vi "Main.vi"(11 "Module Admin":refnum<class "Delacor_lib_QMH_Module Admin.lvclass">) -> ()   [LabVIEW 2021, in "Caption Property Panel.lvlib"]
doc: "This template is based off of the Queued Message Handler design pattern and the Queued Message Handler project template that ships with LabVIEW.\n\nThe main difference is that the queue is private to this module and communication between modules is performed via Broadcast and Request events.\n\nRequest events are wrapped in public API methods and are handled in the Event Handling Loop (EHL) of this VI. Any module can register for Broadcast events sent by this module. The EHL generates messages based on user interface actions.\n\nThe Message Handling Loop (MHL) processes messages generated by the EHL, or by other messages. The messages are string values, so new messages can be added easily to the Message Cases case structure in the MHL. Each message cluster can also provide an optional value for Message Data, which is a variant that can be converted to whatever message-specific data is required.\n_____\nBased on DQMH Project Template 6.0.0.91."
uses:
  Caption Property Panel.lvlib
  <vilib>/Delacor/Delacor QMH/Libraries/Module Admin_class/Delacor_lib_QMH_Module Admin.lvclass
  Module Data--cluster.ctl
  <vilib>/Delacor/Delacor QMH/Libraries/Message Queue_class/Delacor_lib_QMH_Message Queue.lvclass/Delacor_lib_QMH_Message Queue.ctl
  Stop Argument--cluster.ctl
  <vilib>/Delacor/Delacor QMH/Libraries/Module Admin_class/Delacor_lib_QMH_Module Admin.lvclass/Delacor_lib_QMH_Module Admin.ctl
  Initialize Property Value Argument--cluster.ctl
  Load Panel Argument--cluster.ctl
  <vilib>/Utility/miscctls.llb/LVPointTypeDef.ctl
  <vilib>/Delacor/Delacor QMH/Libraries/Message Queue_class/Delacor_lib_QMH_Enqueue Message (Single).vi
  <vilib>/Delacor/Delacor QMH/Libraries/Module Admin_class/Delacor_lib_QMH_Get External Launch.vi
  <vilib>/Utility/error.llb/Error Cluster From Error Code.vi
  <vilib>/ErrorRing/Error Ring.xnode
  <vilib>/Delacor/Delacor QMH/Libraries/Message Queue_class/Delacor_lib_QMH_Message Queue.lvclass
panel:
  in  "Caption":string
  out "error out":errorcluster
  out "Status":string
  in  "Simulate MHL Error":bool
  in  "Simulate EHL Error":bool
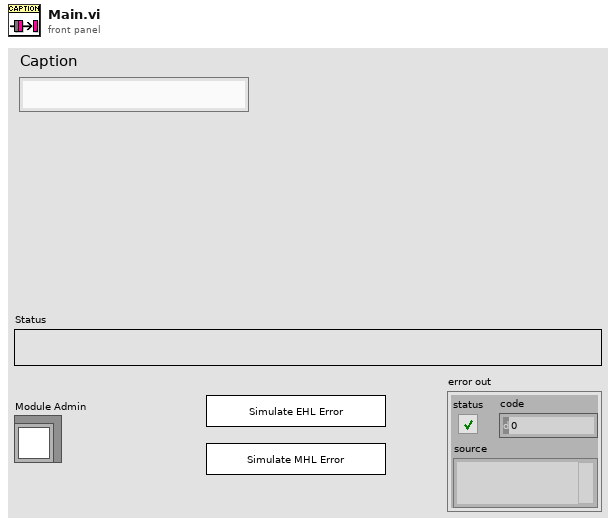
[diagram p1: front panel]
types:
  T1 = typedef "Caption Property Panel.lvlib/Request Events--cluster.ctl" = cluster{"Stop Module":refnum<user-event>, "Show Panel":refnum<user-event>, "Hide Panel":refnum<user-event>, "Get Module Execution Status":refnum<user-event>, "Show Diagram":refnum<user-event>, "Initialize Property Value":refnum<user-event>, "Load Panel":refnum<user-event>}
  T2 = typedef "Caption Property Panel.lvlib/Module Data--cluster.ctl" = cluster{"Status":string}
  T3 = enum32{"invalid lock state", "Not Locked", "Locked (No Password)", "Password-protected"}
  T4 = typedef "Caption Property Panel.lvlib/Stop Argument--cluster.ctl" = cluster{"Origin":string, "Exit via Stop Module Req?":bool, "Wait for Module to stop?":bool}
  T5 = typedef "Caption Property Panel.lvlib/Initialize Property Value Argument--cluster.ctl" = cluster{"Property values":variant[]}
  T6 = typedef "Caption Property Panel.lvlib/Load Panel Argument--cluster.ctl" = cluster{"SubPnl Refnum":refnum<vi>}
  T7 = typedef "LVPointTypeDef.ctl" = cluster{"Horizontal":i16, "Vertical":i16}
  T8 = enum32{"Invalid", "Standard", "Closed", "Hidden", "Minimized", "Maximized"}
  T9 = cluster{"Property value":string, "Variant data":variant}
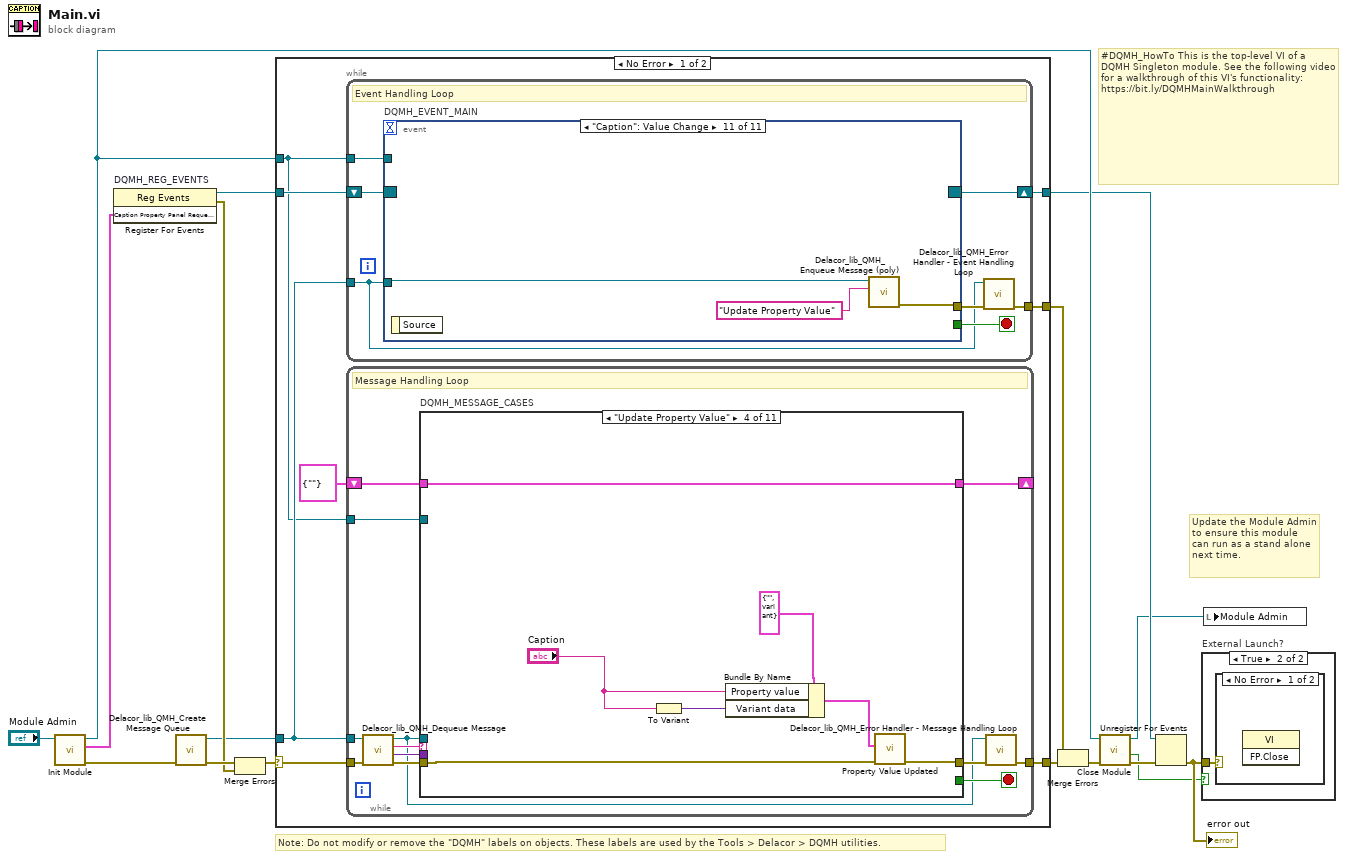
[diagram p0: block diagram]
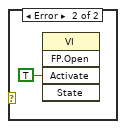
[diagram p3: hidden frame]
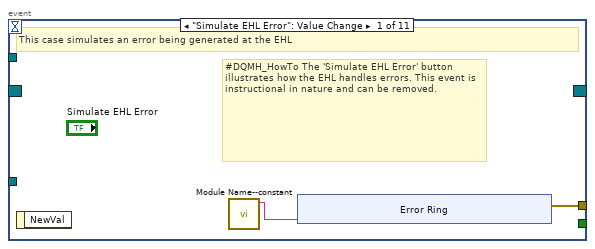
[diagram p4: hidden frame]
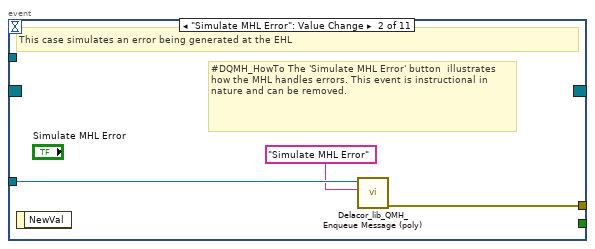
[diagram p5: hidden frame]
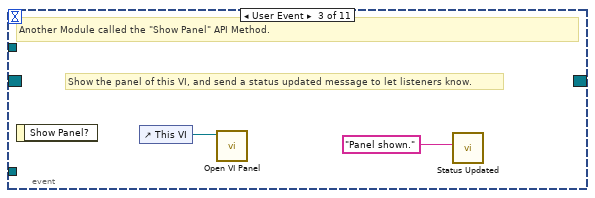
[diagram p6: hidden frame]
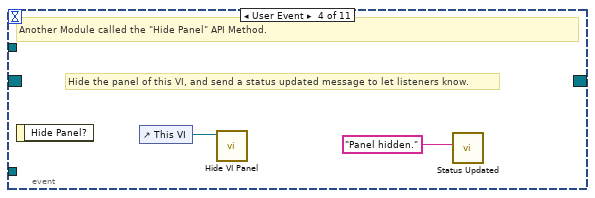
[diagram p7: hidden frame]
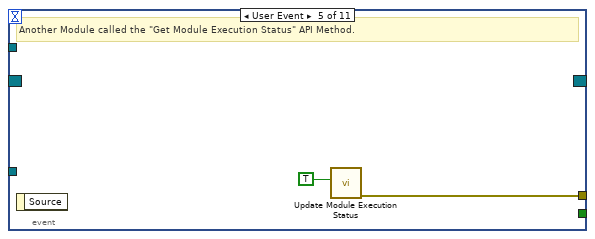
[diagram p8: hidden frame]
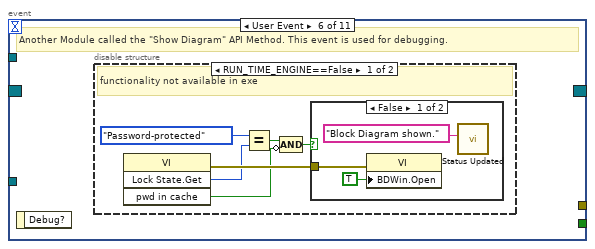
[diagram p9: hidden frame]
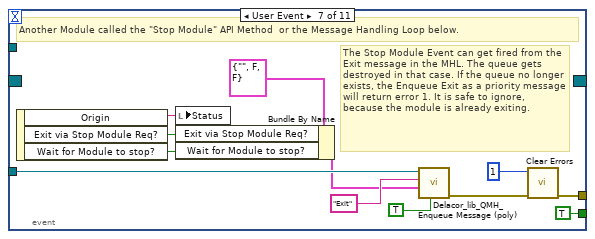
[diagram p12: hidden frame]
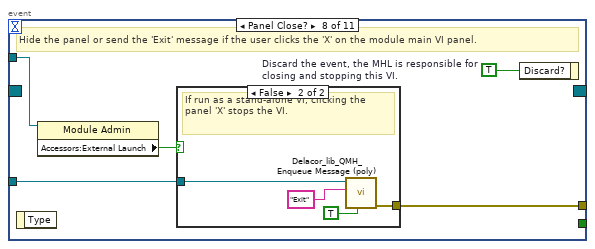
[diagram p13: hidden frame]
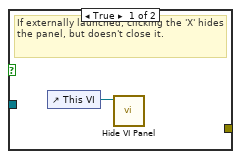
[diagram p14: hidden frame]
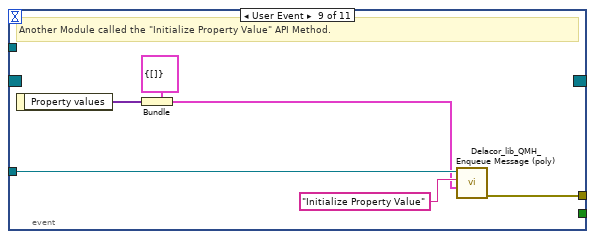
[diagram p15: hidden frame]
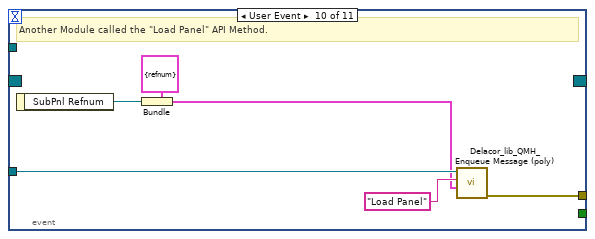
[diagram p16: hidden frame]
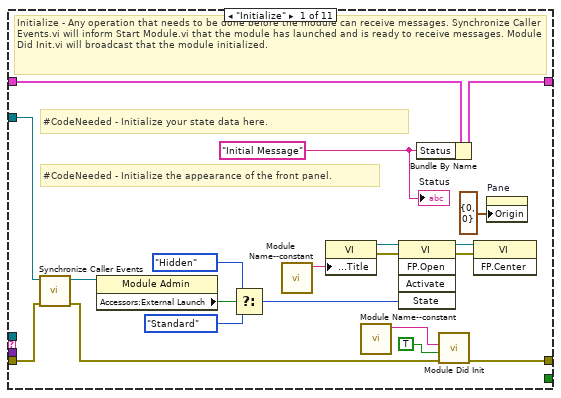
[diagram p17: hidden frame]
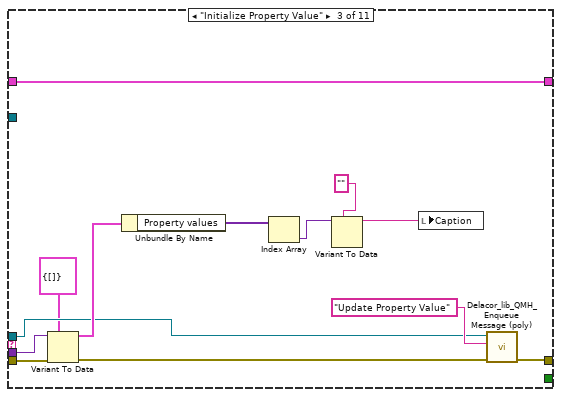
[diagram p19: hidden frame]
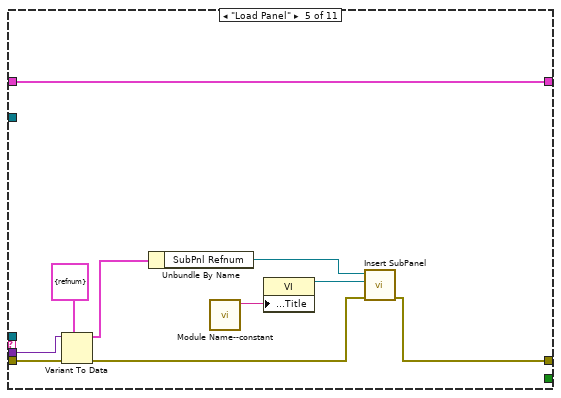
[diagram p20: hidden frame]
diagram:
  # "#DQMH_HowTo This is the top-level VI of a DQMH Singleton module. See the following video for a walkthrough of this VI's functionality: https://bit.ly/DQMHMainWalkthrough"
  # "Note: Do not modify or remove the \"DQMH\" labels on objects. These labels are used by the Tools > Delacor > DQMH utilities."
  # "Update the Module Admin to ensure this module can run as a stand alone next time."
  n1 = call "Init Module.vi"("Singleton Module Admin in"="Module Admin") -> ("error out"=w16:errorcluster, "Caption Property Panel Request Events"=w5:T1, "Singleton Module Admin out"=w8:refnum<class "Delacor_lib_QMH_Module Admin.lvclass">)  [unwired: 8 in]
  n2 = register-events "DQMH_REG_EVENTS"(w5) -> (reference out=w6:refnum<event-registration>, error out=w9:errorcluster)  [unwired: 2 in]
  n3 = call <vilib>:"Delacor_lib_QMH_Create Message Queue.vi"("error in"=w16) -> ("error out"=w11:errorcluster, "Message Queue"=w4:refnum<class "Delacor_lib_QMH_Message Queue.lvclass">)  [unwired: 9 in]
  n4 = Merge Errors(w11, w9) -> (w10:errorcluster)
  n5 = case shown="No Error" w10 {
    selector: w10 -> [w23 w225]
    tunnel: [w25 w224] -> w17
    tunnel: [w22 w230] -> w7
    tunnel: w6 -> [w20 w230]
    tunnel: w4 -> [w19 w223]
    tunnel: [w24 _] -> w14
    tunnel: w8 -> [w18 w226]
    frame No Error {
      n6 = while {
        tunnel: w19 -> [w26]
        shift-right: [w29] -> w22
        shift-left: w20 -> [w30]
        tunnel: [w31] -> w24
        tunnel: w18 -> [w27]
        stop <- w28 stop-if-true
        # "Event Handling Loop"
        n7 = event "DQMH_EVENT_MAIN" shown="[10] \"Caption\": Value Change" {
          selector: w30 -> [_ _ _ _ _ _ _ _ _ _ _]
          dyn-events: [_ _ _ _ _ _ _ _ _ _ _] -> w29
          timeout: _ -> [_ _ _ _ _ _ _ _ _ _ _]
          tunnel: [_ _ _ _ _ _ TRUE ("Discard?") _ _ _ _] -> w28
          tunnel: w26 -> [_ w43 _ _ _ _ w67 w74 w87 w93 w94]
          tunnel: [w34 w44 _ _ w50 _ w70 w76 w82 w88 w95] -> w32
          tunnel: w27 -> [_ _ _ _ _ _ _ w73 _ _ _]
          event "Simulate EHL Error": Value Change {
            # "#DQMH_HowTo The 'Simulate EHL Error' button  illustrates how the EHL handles errors. This event is instructional in nature and can be removed."
            # "This case simulates an error being generated at the EHL"
            n8 = event-data() -> ()  [unwired: 1 in, 1 out]
            n9 = call "Module Name--constant.vi"() -> ("Module Name"=w33:string)  [unwired: 11 in]
            n10 = xnode "Error Ring"("parameter 0"=w33) -> ("error out"=w34:errorcluster)
          }
          event "Simulate MHL Error": Value Change {
            # "#DQMH_HowTo The 'Simulate MHL Error' button  illustrates how the MHL handles errors. This event is instructional in nature and can be removed."
            # "This case simulates an error being generated at the EHL"
            n11 = event-data() -> ()  [unwired: 1 in, 1 out]
            n12 = call-poly <vilib>:"Delacor_lib_QMH_Enqueue Message (poly).vi"("Message"="Simulate MHL Error", "Message Queue in"=w43) -> ("error out"=w44:errorcluster)  [unwired: 8 in, 1 out]
          }
          event User Event {
            # "Show the panel of this VI, and send a status updated message to let listeners know."
            # "Another Module called the \"Show Panel\" API Method."
            n13 = event-data() -> ()  [unwired: 1 in, 1 out]
            n14 = control-ref of="This VI"() -> (w46:refnum<vi>)
            n15 = call "Open VI Panel.vi"("VI"=w46) -> ()  [unwired: 10 in, 1 out]
            n16 = call "Status Updated.vi"("Status"="Panel shown." ("format string")) -> ()  [unwired: 10 in, 1 out]
          }
          event User Event {
            # "Hide the panel of this VI, and send a status updated message to let listeners know."
            # "Another Module called the \"Hide Panel\" API Method."
            n17 = event-data() -> ()  [unwired: 1 in, 1 out]
            n18 = control-ref of="This VI"() -> (w48:refnum<vi>)
            n19 = call "Hide VI Panel.vi"("VI"=w48) -> ()  [unwired: 10 in, 1 out]
            n20 = call "Status Updated.vi"("Status"="Panel hidden." ("format string")) -> ()  [unwired: 10 in, 1 out]
          }
          event User Event {
            # "Another Module called the \"Get Module Execution Status\" API Method."
            n21 = event-data() -> ()  [unwired: 1 in, 1 out]
            n22 = call "Update Module Execution Status.vi"("Running?"=TRUE) -> ("error out"=w50:errorcluster)  [unwired: 10 in]
          }
          event User Event {
            # "Another Module called the \"Show Diagram\" API Method. This event is used for debugging."
            n23 = event-data() -> ()  [unwired: 1 in, 1 out]
            n24 = disable-structure shown="RUN_TIME_ENGINE==False" {
              frame condition #0 (active) {
                # "functionality not available in exe"
                n25 = invoke class="VI" method="Lock State.Get"() -> (error out=w56:errorcluster, "Get Lock State"=w55:T3, "pwd in cache"=w52:bool)  [unwired: 4 in, 1 out]
                n26 = Equal?(x=T3."Password-protected", y=w55) -> (x = y?=w53:bool)
                n27 = Compound Arithmetic op=AND(w53, invert w52) -> (w51:bool)
                n28 = case shown="False" w51 {
                  tunnel: w56 -> [w59 _]
                  frame False {
                    n29 = property class="VI"(error in=w59, "BDWin.Open"=TRUE ("Block Diagram Window:Open")) -> ()  [unwired: 1 in, 2 out]
                    n30 = call "Status Updated.vi"("Status"="Block Diagram shown." ("format string")) -> ()  [unwired: 10 in, 1 out]
                  }
                  frame True {
                    # "Password-protected VI, and the password is not in the cache. Do not show the diagram."
                  }
                }
              }
              frame condition #1 {
              }
            }
          }
          event User Event {
            # "The Stop Module Event can get fired from the Exit message in the MHL. The queue gets destroyed in that case. If the queue no longer exists, the Enqueue Exit as a priority message will return error 1. It is safe to ignore, because the module is already exiting."
            # "Another Module called the \"Stop Module\" API Method  or the Message Handling Loop below."
            n31 = event-data() -> ("Origin"=w66:string, "Exit via Stop Module Req?"=w62:bool, "Wait for Module to stop?"=w61:bool)  [unwired: 1 in]
            n32 = local write "Status"(w66) -> ()
            n33 = Bundle By Name(cluster=T4 {"Origin"="", "Exit via Stop Module Req?"=FALSE, "Wait for Module to stop?"=FALSE} ("Stop Argument"), "Exit via Stop Module Req?"=w62, "Wait for Module to stop?"=w61) -> (w60:T4)
            n34 = call-poly <vilib>:"Delacor_lib_QMH_Enqueue Message (poly).vi"("Priority Message? (F)"=TRUE, "Message Data"=w60, "Message"="Exit", "Message Queue in"=w67) -> ("error out"=w71:errorcluster)  [unwired: 6 in, 1 out]
            n35 = call <vilib>:"Clear Errors.vi"("error in (no error)"=w71, "specific error code to clear (0: all)"=1) -> ("error out"=w70:errorcluster)  [unwired: 4 in, 1 out]
          }
          event Panel Close? {
            w75 = TRUE  # Discard the event, the MHL is responsible for closing and stopping this VI.
            # "Hide the panel or send the 'Exit' message if the user clicks the 'X' on the module main VI panel."
            n36 = event-data() -> ()  [unwired: 1 in, 1 out]
            n37 = property class="Module Admin"(reference=w73) -> ("Accessors:External Launch"=w72:bool)  [unwired: 1 in, 2 out]
            n38 = case shown="False" w72 {
              tunnel: w74 -> [_ w80]
              tunnel: [_ w81] -> w76
              frame True {
                # "If externally launched, clicking the 'X' hides the panel, but doesn't close it."
                n39 = control-ref of="This VI"() -> (w77:refnum<vi>)
                n40 = call "Hide VI Panel.vi"("VI"=w77) -> ()  [unwired: 10 in, 1 out]
              }
              frame False {
                # "If run as a stand-alone VI, clicking the panel 'X' stops the VI."
                n41 = call-poly <vilib>:"Delacor_lib_QMH_Enqueue Message (poly).vi"("Priority Message? (F)"=TRUE, "Message"="Exit", "Message Queue in"=w80) -> ("error out"=w81:errorcluster)  [unwired: 7 in, 1 out]
              }
            }
            n42 = event-data("Discard?"=w75) -> ()  [unwired: 1 in, 1 out]
          }
          event User Event {
            # "Another Module called the \"Initialize Property Value\" API Method."
            n43 = event-data() -> ("Property values"=w83:variant[])  [unwired: 1 in]
            n44 = Bundle(cluster=T5 {"Property values"=[]} ("Initialize Property Value Argument"), "Property values"=w83) -> (w84:T5)
            n45 = call-poly <vilib>:"Delacor_lib_QMH_Enqueue Message (poly).vi"("Message Data"=w84, "Message"="Initialize Property Value", "Message Queue in"=w87) -> ("error out"=w82:errorcluster)  [unwired: 7 in, 1 out]
          }
          event User Event {
            # "Another Module called the \"Load Panel\" API Method."
            n46 = event-data() -> ("SubPnl Refnum"=w89:refnum<vi>)  [unwired: 1 in]
            n47 = Bundle(cluster=T6 {"SubPnl Refnum"=refnum} ("Load Panel Argument"), "SubPnl Refnum"=w89) -> (w90:T6)
            n48 = call-poly <vilib>:"Delacor_lib_QMH_Enqueue Message (poly).vi"("Message Data"=w90, "Message"="Load Panel", "Message Queue in"=w93) -> ("error out"=w88:errorcluster)  [unwired: 7 in, 1 out]
          }
          event "Caption": Value Change {
            n49 = event-data() -> ()  [unwired: 1 in, 1 out]
            n50 = call-poly <vilib>:"Delacor_lib_QMH_Enqueue Message (poly).vi"("Message"="Update Property Value", "Message Queue in"=w94) -> ("error out"=w95:errorcluster)  [unwired: 8 in, 1 out]
          }
        }
        n51 = call-dynamic "Delacor_lib_QMH_Error Handler - Event Handling Loop.vi"("error in"=w32, "Message Queue in"=w26) -> ("dup error in"=w31:errorcluster)  [unwired: 8 in, 1 out]
      }
      n52 = while {
        tunnel: w19 -> [w99]
        shift-right: [w103] -> _
        shift-left: T2 {"Status"=""} ("Data Cluster") -> [w104]
        tunnel: w23 -> [w107]
        tunnel: [w105] -> w25
        tunnel: w18 -> [w97]
        stop <- w102 stop-if-true
        # "Message Handling Loop"
        n53 = call-dynamic "Delacor_lib_QMH_Dequeue Message.vi"("error in"=w107, "Message Queue in"=w99) -> ("error out"=w106:errorcluster, "Message Data"=w100:variant, "Message"=w101:string, "Message Queue out"=w98:refnum<class "Delacor_lib_QMH_Message Queue.lvclass">)  [unwired: 6 in]
        n54 = case "DQMH_MESSAGE_CASES" shown="\"Update Property Value\"" w101 {
          selector: w101 -> [_ _ _ _ _ _ _ _ _ _ w210]
          tunnel: w98 -> [_ _ w133 _ _ _ _ _ w180 w202 _]
          tunnel: w106 -> [w126 w130 w135 w147 w155 w163 w165 w170 w187 w208 w212]
          tunnel: [w124 w130 w132 w146 w153 w162 w165 w169 w183 w205 w213] -> w108
          tunnel: w104 -> [w115 w129 w143 w150 w160 w161 w164 w167 w182 w201 w211]
          tunnel: [w114 w129 w143 w150 w160 w161 w164 w167 w182 w201 w211] -> w103
          tunnel: [_ _ _ _ _ _ _ _ _ w200 _] -> w102
          tunnel: w100 -> [_ _ w134 _ w154 _ _ _ w181 w199 _]
          tunnel: w97 -> [w116 _ _ _ _ _ _ _ w179 w194 _]
          frame "Initialize" {
            w110 = "Initial Message" ("Initial Message")
            # "#CodeNeeded - Initialize the appearance of the front panel."
            # "#CodeNeeded - Initialize your state data here."
            # "Initialize - Any operation that needs to be done before the module can receive messages. Synchronize Caller Events.vi will inform Start Module.vi that the module has launched and is ready to receive messages. Module Did Init.vi will broadcast that the module initialized."
            n55 = call "Synchronize Caller Events.vi"("error in (no error)"=w126, "Singleton Module Admin in"=w116) -> ("error out"=w125:errorcluster, "Singleton Module Admin out"=w111:refnum<class "Delacor_lib_QMH_Module Admin.lvclass">)  [unwired: 8 in]
            n56 = property class="Module Admin"(reference=w111) -> ("Accessors:External Launch"=w120:bool)  [unwired: 1 in, 2 out]
            n57 = Select(t=T8."Hidden" ("State"), s=w120, f=T8."Standard" ("State")) -> (s? t:f=w117:T8)
            n58 = call "Module Name--constant.vi"() -> ("Module Name"=w123:string)  [unwired: 11 in]
            n59 = property class="VI"("Front Panel.Title"=w123) -> (reference out=w122:refnum<vi>, error out=w128:errorcluster)  [unwired: 2 in]
            n60 = call "Module Name--constant.vi"() -> ("Module Name"=w112:string)  [unwired: 11 in]
            n61 = invoke class="VI" method="FP.Open"(reference=w122, error in=w128, "State"=w117) -> (reference out=w121:refnum<vi>, error out=w127:errorcluster)  [unwired: 2 in, 3 out]
            n62 = Bundle By Name(cluster=w115, "Status"=w110) -> (w114:T2)
            n63 = call "Module Did Init.vi"("error in (no error)"=w125, "Initialized?"=TRUE, "Origin"=w112) -> ("error out"=w124:errorcluster)  [unwired: 8 in]
            n64 = invoke class="VI" method="FP.Center"(reference=w121, error in=w127) -> ()  [unwired: 1 in, 3 out]
            n65 = property on="Pane" class="Pane"("Origin"=T7 {"Horizontal"=0, "Vertical"=0}) -> ()  [unwired: 2 in, 2 out]
            "Status" <- w110
          }
          frame "---Module Specific---" {
            # "Separator -- The following cases handle messages specific to this Module."
          }
          frame "Initialize Property Value" {
            n66 = Variant To Data(error in=w135, type=T5 {"Property values"=[]} ("Initialize Property Value Argument"), Variant=w134) -> (data=w138:T5, error out=w139:errorcluster)
            n67 = Unbundle By Name(w138) -> ("Property values"=w140:variant[])
            n68 = Index Array(array=w140) -> (element=w141:variant)  [unwired: 1 in]
            n69 = Variant To Data(type="", Variant=w141) -> (data=w142:string)  [unwired: 1 in, 1 out]
            n70 = local write "Caption"(w142) -> ()
            n71 = call-poly <vilib>:"Delacor_lib_QMH_Enqueue Message (poly).vi"("error in"=w139, "Message"="Update Property Value", "Message Queue in"=w133) -> ("error out"=w132:errorcluster)  [unwired: 7 in, 1 out]
          }
          frame "Update Property Value" {
            n72 = To Variant(anything="Caption") -> (Variant=w148:variant)
            n73 = Bundle By Name(cluster=T9 {"Property value"="", "Variant data"=variant} ("Property data"), "Property value"="Caption", "Variant data"=w148) -> (w145:T9)
            n74 = call "Property Value Updated.vi"("error in"=w147, "Property data"=w145) -> ("error out"=w146:errorcluster)  [unwired: 9 in]
          }
          frame "Load Panel" {
            n75 = Variant To Data(error in=w155, type=T6 {"SubPnl Refnum"=refnum} ("Load Panel Argument"), Variant=w154) -> (data=w159:T6, error out=w156:errorcluster)
            n76 = Unbundle By Name(w159) -> ("SubPnl Refnum"=w158:refnum<vi>)
            n77 = call "Module Name--constant.vi"() -> ("Module Name"=w152:string)  [unwired: 11 in]
            n78 = property on="Property Node" class="VI"("Front Panel.Title"=w152) -> (reference out=w157:refnum<vi>)  [unwired: 2 in, 1 out]
            n79 = call "Insert SubPanel.vi"("error in (no error)"=w156, "VI Ref"=w157, "Subpanel Ref"=w158) -> ("error out"=w153:errorcluster)  [unwired: 8 in]
          }
          frame "---Copy This Frame---" {
            # "Duplicate this frame when creating new messages.  Change this comment in the duplicated frame to describe this message."
            n80 = Merge Errors(w163) -> (w162:errorcluster)
          }
          frame "---Exit and Error Handling---" {
            # "Separator - The following cases handle errors and exit messages."
          }
          frame "Simulate MHL Error" {
            # "#DQMH_HowTo The 'Simulate MHL Error' button  illustrates how the MHL handles errors. This event is instructional in nature and can be removed."
            # "Simulate an error occurring at the MHL"
            n81 = call "Module Name--constant.vi"() -> ("Module Name"=w166:string)  [unwired: 11 in]
            n82 = xnode "Error Ring"("parameter 0"=w166) -> ("error out"=w168:errorcluster)
            n83 = Merge Errors(w170, w168) -> (w169:errorcluster)
          }
          frame "Error" {
            # "#CodeRecommended - If you ever change the name of this \"Error\" message, you'll need to update the name in the Check Loop Error.vi as well."
            # "#CodeRecommended - If the module is running in standalone mode (External Launch = FALSE), this code will pop up an error dialog and call the 'Exit' message if an error occurs. Add more fine-grained error handling here."
            # "Error - Check the error message data and respond accordingly. This message is sent by the \"Error Handler\" VIs at the end of each loop in this application."
            n84 = property class="Module Admin"(reference=w179) -> ("Accessors:External Launch"=w178:bool)  [unwired: 1 in, 2 out]
            n85 = Variant To Data(error in=w187, type=errorcluster {"status"=FALSE, "code"=0, "source"=""} ("error constant"), Variant=w181) -> (data=w188:errorcluster, error out=w185:errorcluster)
            n86 = call "Error Reported.vi"("Error"=w188) -> ()  [unwired: 10 in, 1 out]
            n87 = case shown="False" w178 {
              tunnel: [w193 _] -> w184
              tunnel: w180 -> [w191 _]
              tunnel: w188 -> [w192 _]
              frame False {
                # "If the module is running standalone, then pop up an error dialog and call the \"Exit\" message."
                n88 = call <vilib>:"Simple Error Handler.vi"("error in (no error)"=w192) -> ()  [unwired: 4 in, 5 out]
                n89 = call-poly <vilib>:"Delacor_lib_QMH_Enqueue Message (poly).vi"("Priority Message? (F)"=TRUE, "Message"="Exit", "Message Queue in"=w191) -> ("error out"=w193:errorcluster)  [unwired: 7 in, 1 out]
              }
              frame True {
                # "If the module was launched externally, calling the Error Reported broadcast VI is the only action performed by the \"Error\" message. The module's caller can then process the error appropriately."
              }
            }
            n90 = Merge Errors(w185, w184) -> (w183:errorcluster)
            n91 = local write "error out"(w183) -> ()
          }
          frame "Exit" {
            w198 = 91  # 91: not all Exit messages will have an argument
            w200 = TRUE  # Stop the VI
            # "Release the message queue reference"
            # "#CodeNeeded - Add any required cleanup code here"
            # "Exit - Exit the application."
            n92 = Variant To Data(error in=w208, type=T4 {"Origin"="", "Exit via Stop Module Req?"=FALSE, "Wait for Module to stop?"=FALSE} ("Stop Argument"), Variant=w199) -> (data=w196:T4, error out=w204:errorcluster)
            n93 = call <vilib>:"Clear Errors.vi"("error in (no error)"=w204, "specific error code to clear (0: all)"=w198) -> ("error out"=w207:errorcluster)  [unwired: 4 in, 1 out]
            n94 = control-ref of="This VI"() -> (w195:refnum<vi>)
            n95 = call-dynamic "Delacor_lib_QMH_Release Message Queue.vi"("error in"=w207, "Message Queue"=w202) -> ("error out"=w206:errorcluster)  [unwired: 9 in]
            n96 = call "Handle Exit.vi"("Stop Argument"=w196, "Admin in"=w194, "VI reference"=w195) -> ("error out"=w203:errorcluster)  [unwired: 7 in, 1 out]
            n97 = Merge Errors(w206, w203) -> (w205:errorcluster)
          }
          frame Default {
            # "'Default' case only runs if there is a message that isn't defined in any of the other cases.  Output a programming error."
            n98 = call "Module Name--constant.vi"() -> ("Module Name"=w209:string)  [unwired: 11 in]
            n99 = xnode "Error Ring"("parameter 0"=w210, "parameter 1"=w209) -> ("error out"=w214:errorcluster)
            n100 = Merge Errors(w212, w214) -> (w213:errorcluster)
          }
        }
        n101 = call-dynamic "Delacor_lib_QMH_Error Handler - Message Handling Loop.vi"("error in"=w108, "Message Queue in"=w98) -> ("dup error in"=w105:errorcluster)  [unwired: 8 in, 1 out]
      }
    }
    frame Error {
      # "Synchronize Caller Events.vi will inform Start Module.vi that the module has launched and will let the code calling Start Module.vi register for broadcasts and would permit the caller receive the broadcast that an error occurred at launch time."
      n102 = call-dynamic "Delacor_lib_QMH_Release Message Queue.vi"("error in"=w225, "Message Queue"=w223) -> ("error out"=w224:errorcluster)  [unwired: 9 in]
      n103 = call "Synchronize Caller Events.vi"("Singleton Module Admin in"=w226) -> ("error out"=w231:errorcluster)  [unwired: 9 in, 1 out]
      n104 = call "Module Name--constant.vi"() -> ("Module Name"=w229:string)  [unwired: 11 in]
      n105 = Format Into String(format string="An error occurred during initialization. %s is no longer running.", w229) -> (resulting string=w227:string)  [unwired: 2 in, 1 out]
      n106 = Merge Errors(w224, w231) -> (w232:errorcluster)
      n107 = call "Error Reported.vi"("Additional Information"=w227, "Error"=w232) -> ()  [unwired: 9 in, 1 out]
    }
  }
  n108 = Merge Errors(w14, w17) -> (w13:errorcluster)
  n109 = call "Close Module.vi"("error in (no error)"=w13, "Module Admin in"=w8) -> ("error out"=w15:errorcluster, "External Launch"=w1:bool, "Module Admin out"=w2:refnum<class "Delacor_lib_QMH_Module Admin.lvclass">)  [unwired: 7 in]
  n110 = Unregister For Events(event registration refnum=w7, error in=w15) -> (error out=w12:errorcluster)
  "error out" <- w12
  n111 = case "External Launch?" shown="True" w1 {
    tunnel: w12 -> [_ w233]
    frame False {
    }
    frame True {
      n112 = case shown="No Error" w233 {
        frame No Error {
          n113 = invoke class="VI" method="FP.Close"() -> ()  [unwired: 3 in, 3 out]
        }
        frame Error {
          n114 = invoke class="VI" method="FP.Open"("Activate"=TRUE ("Activate?")) -> ()  [unwired: 4 in, 5 out]
        }
      }
    }
  }
  n115 = local write "Module Admin"(w2) -> ()
